vi "DB_CONFIGURATION.vi"(9 "TYPE ?":bool, 10 "PRODUCTS":T1, 11 "MONEY":T2) -> (2 "created":bool, 3 "avaiable":bool)   [LabVIEW 2019]
uses:
  Libraries/DB_VENDING MACHINE/Type Defs/MONEY.ctl
  Libraries/DB_VENDING MACHINE/Type Defs/PRODUCTS.ctl
  Libraries/DB_VENDING MACHINE/DB_VENDING MACHINE.lvlib
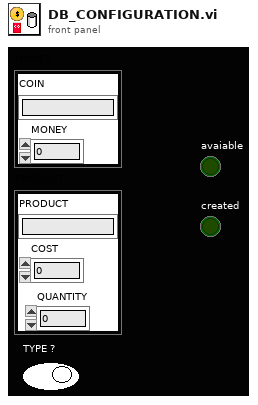
[diagram p1: front panel]
types:
  T1 = typedef "DB_VENDING MACHINE.lvlib/PRODUCTS.ctl" = cluster{"PRODUCT":string, "COST":dbl, "QUANTITY":i8}
  T2 = typedef "DB_VENDING MACHINE.lvlib/MONEY.ctl" = cluster{"COIN":string, "MONEY":dbl}
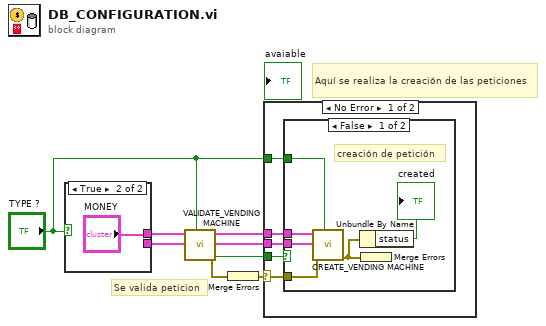
[diagram p0: block diagram]
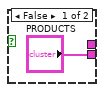
[diagram p2: hidden frame]
diagram:
  # "Se valida peticion"
  # "Aquí se realiza la creación de las peticiones"
  n1 = case shown="True" "TYPE ?" {
    tunnel: [_ "MONEY"] -> w5
    tunnel: ["PRODUCTS" _] -> w4
    frame False {
    }
    frame True {
    }
  }
  n2 = call "VALIDATE_VENDING MACHINE.vi"("TYPE ?"="TYPE ?", "PRODUCTS"=w4, "MONEY"=w5) -> ("error out"=w7:errorcluster, "Valido?"=w2:bool, "PRODUCTS OUT"=w3:T1, "MONEY OUT"=w6:T2)  [unwired: 5 in]
  n3 = Merge Errors(w7) -> (w8:errorcluster)
  n4 = case shown="No Error" w8 {
    selector: w8 -> [w15 _]
    tunnel: w6 -> [w14 _]
    tunnel: w3 -> [w13 _]
    tunnel: w2 -> [w12 _]
    tunnel: "TYPE ?" -> [w11 _]
    frame No Error {
      n5 = case shown="False" w12 {
        tunnel: w15 -> [w20 _]
        tunnel: w14 -> [w18 _]
        tunnel: w13 -> [w17 _]
        tunnel: w11 -> [w16 _]
        frame False {
          # "creación de petición"
          n6 = call "CREATE_VENDING MACHINE.vi"("TYPE ?"=w16, "error in (no error)"=w20, "PRODUCTS"=w17, "MONEY"=w18) -> ("error out"=w21:errorcluster)  [unwired: 7 in]
          n7 = Unbundle By Name(w21) -> ("status"=→"created":bool)
          n8 = Merge Errors(w21) -> ()  [unwired: 1 out]
        }
        frame True {
        }
      }
    }
    frame Error {
    }
  }
